vi "demod_low.vi"(0 "Reset":bool, 5 "Config":T5={"I/O"={"Format"={"Rate"=4, "Bits"=32, "Channels"=2}, "card #"=1, "# buffers"=96000}, "High rate STFT"={"Win param"=101.5, "Window type"=61, "Win order"=2, "DFT size"=64, "Channels"=[7], "Oversample"=64}, "Low rate STFT"={"Win param"=120.0, "Window type"=61, "Win order"=8, "DFT size"=64, "Channels"=[7], "Oversample"=64}, "Filtering"={"Hum"={"Frequency"=0.0, "Tc"=0.0, "Limit"=101.5, "FFT filter"=FALSE, "Detrend mode"=enum."Robust linear", "Enable"=FALSE}, "Kalman"={"Process noise"=101.5, "Measure noise"=101.5, "Unlock m noise"=101.5, "Mode"=enum."FFT"}, "Distortion"={"LF cut"=101.5, "Tc"=3.0, "Limit"=101.5, "FFT filter"=FALSE, "Detrend mode"=enum."Robust linear", "Enable"=FALSE}, "Lowpass"={"Frequency"=0.0, "Order"=0, "Enable"=FALSE}, "Impulse"={"Win order"=102, "Locked limit"=101.5, "Locked count"=102, "Threshold Tc"=101.5, "Thresh sigmas"=101.5, "Thresh min"=101.5, "After"=0, "Detrend"=FALSE, "Enable"=FALSE}}} {"Filtering"."Impulse"."Thresh min" format="%#_3p"; "Filtering"."Impulse"."Threshold Tc" format="%#_3p"; "Filtering"."Impulse"."Locked limit" format="%#_3p"; "Filtering"."Impulse"."Thresh sigmas" format="%#_3p"; "Filtering"."Lowpass"."Frequency" format="%#_4p"; "Filtering"."Distortion"."Limit" format="%#_3p"; "Filtering"."Distortion"."LF cut" format="%#_3p"; "Filtering"."Kalman"."Unlock m noise" format="%#_3p"; "Filtering"."Kalman"."Measure noise" format="%#_3p"; "Filtering"."Kalman"."Process noise" format="%#_3p"; "Filtering"."Hum"."Limit" format="%#_3p"; "Filtering"."Hum"."Frequency" format="%#_4p"; "Low rate STFT"."Oversample" min=1 step=1; "Low rate STFT"."Channels" min=0 step=1; "Low rate STFT"."DFT size" min=1 step=1; "Low rate STFT"."Window type" items=["Rectangle"=0, "Hanning"=1, "Hamming"=2, "Blackman-Harris"=3, "Exact Blackman"=4, "Blackman"=5, "Flat Top"=6, "4 Term B-Harris "=7, "7 Term B-Harris"=8, "Low Sidelobe"=9, "Blackman Nuttall"=11, "Triangle"=30, "Bartlett-Hanning"=31, "Bohman"=32, "Parzen"=33, "Welch"=34, "Kaiser"=60, "Dolph-Chebyshev"=61, "Gaussian"=62]; "High rate STFT"."Oversample" min=1 step=1; "High rate STFT"."Channels" min=0 step=1; "High rate STFT"."DFT size" min=1 step=1; "High rate STFT"."Window type" items=["Rectangle"=0, "Hanning"=1, "Hamming"=2, "Blackman-Harris"=3, "Exact Blackman"=4, "Blackman"=5, "Flat Top"=6, "4 Term B-Harris "=7, "7 Term B-Harris"=8, "Low Sidelobe"=9, "Blackman Nuttall"=11, "Triangle"=30, "Bartlett-Hanning"=31, "Bohman"=32, "Parzen"=33, "Welch"=34, "Kaiser"=60, "Dolph-Chebyshev"=61, "Gaussian"=62]}, 7 "Modulation info":T1={"Fs full"=0.0, "Fs high"=0.0, "Fs low"=0.0, "Read size"=0, "FFT size low"=5000, "df low"=5000.0, "High carriers"=[], "Low carriers"=[], "Hi channels at low"=[7]} {"Hi channels at low" min=0 step=1; "Low carriers" format="%#_6p"; "High carriers" format="%#_6p"}, 11 "Trace info in":T2, 12 "Filtered data":dbl[][](array[numeric])) -> (4 "Carrier amplitudes":cdb[][][](array[numeric]) format="%#_3p", 15 "Trace info out":T2)   [LabVIEW 2014]
uses:
  ilemt_config.ctl
  io_config.ctl
  stft_params.ctl
  <vilib>/Analysis/4window.llb/windowTd.ctl
  filter_params.ctl
  detrend_mode.ctl
  trace_info.ctl
  trace_channel.ctl
  ilemt_status.ctl
  modulation_info.ctl
  <vilib>/Analysis/NI_AALPro.lvlib
panel:
  # "Rows are same format as raw data, 3 filtered sensor signals, followed by 3 (not Kalman filtered) current sense inputs."
  # "First dimension (page) selects input channel: sensor X, Y, Z or current sense.  There is only one set of currents even though there are three sense inputs because we only report X magnitude on X, Y on Y, etc., discarding the cross coupling terms."
  # "High"
  # "Low"
  # "X"
  # "Y"
  # "Z"
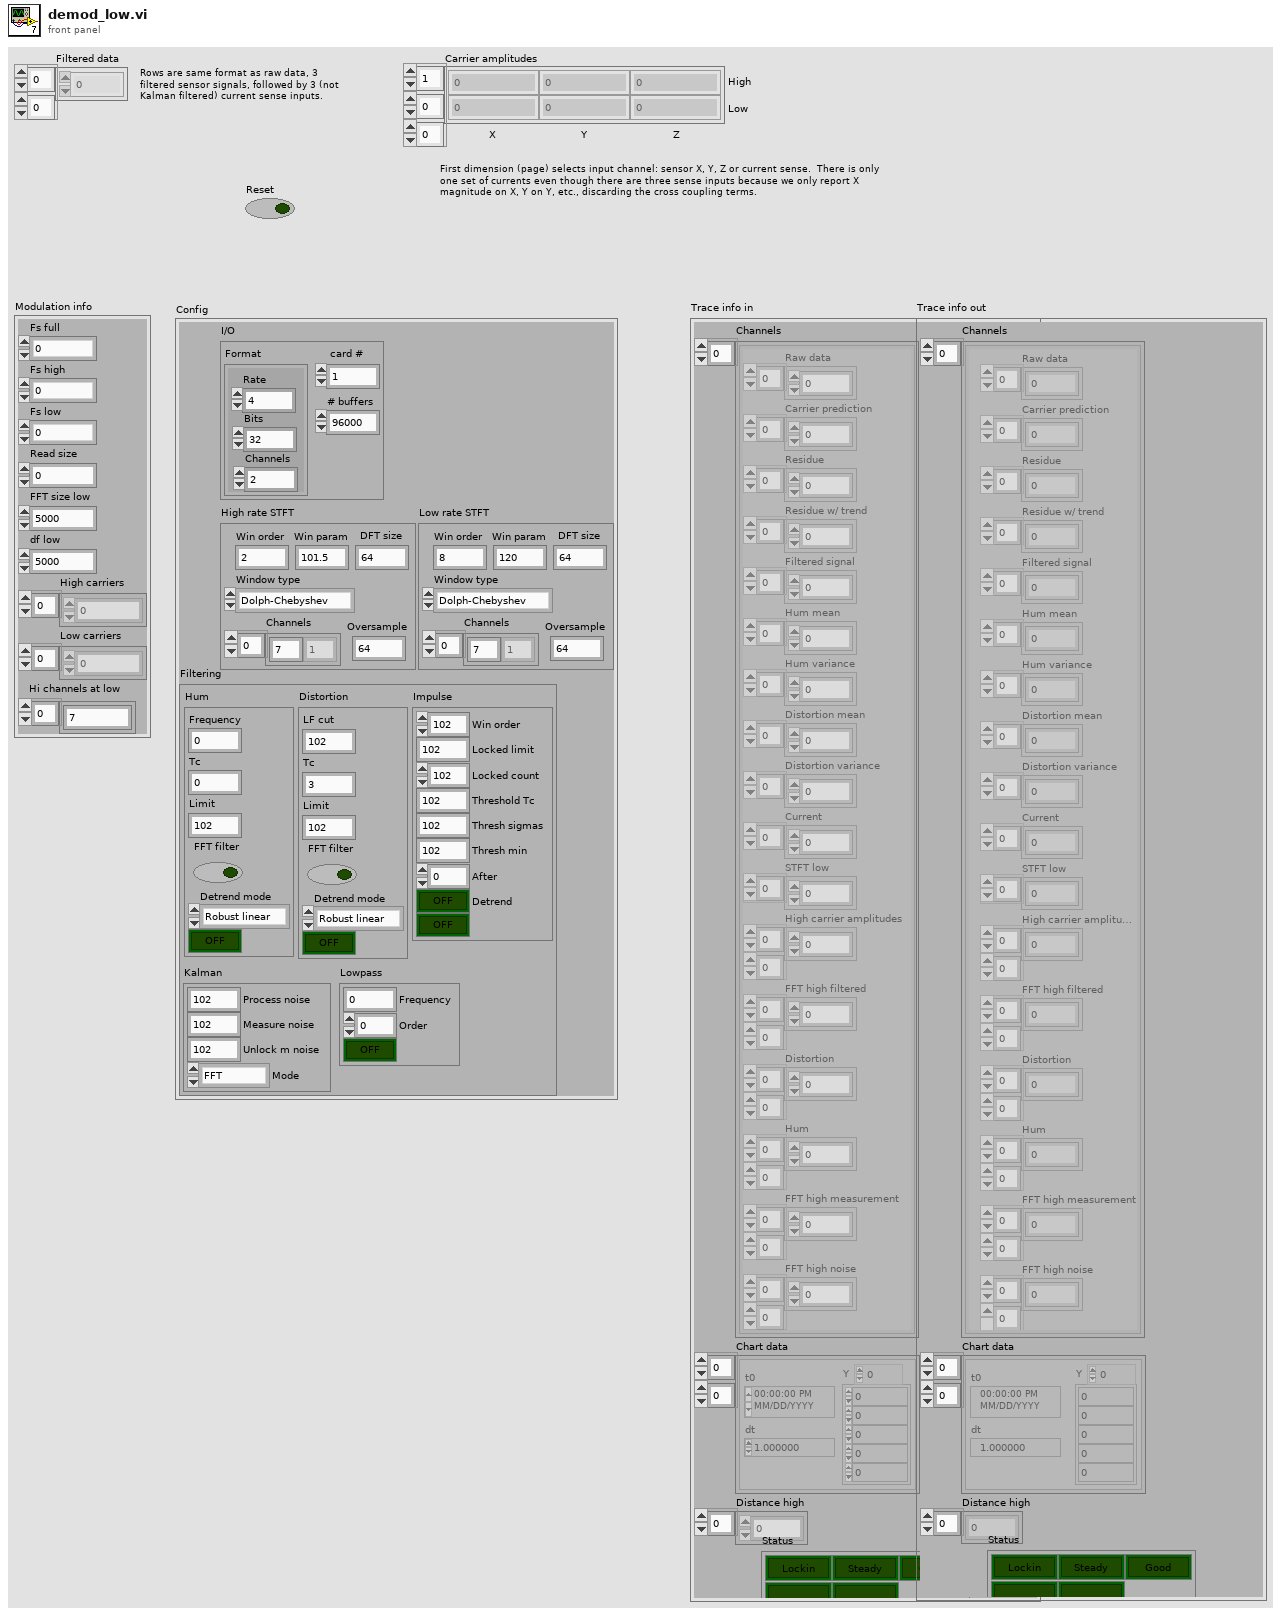
[diagram p1: front panel]
types:
  T1 = typedef "modulation_info.ctl" = cluster{"Fs full":dbl, "Fs high":dbl, "Fs low":dbl, "Read size":i32, "FFT size low":i32, "df low":dbl, "High carriers":dbl[], "Low carriers":dbl[], "Hi channels at low":i32[]}
  T2 = typedef "trace_info.ctl" = cluster{"Channels":T3[], "Chart data":waveform(dbl)[][], "Distance high":dbl[], "Status":T4}
  T3 = typedef "trace_channel.ctl" = cluster{"Raw data":dbl[], "Carrier prediction":dbl[], "Residue":dbl[], "Residue w/ trend":dbl[], "Filtered signal":dbl[], "Hum mean":dbl[], "Hum variance":dbl[], "Distortion mean":dbl[], "Distortion variance":dbl[], "Current":dbl[], "STFT low":cdb[], "High carrier amplitudes":cdb[][], "FFT high filtered":cdb[][], "Distortion":cdb[][], "Hum":cdb[][], "FFT high measurement":cdb[][], "FFT high noise":dbl[][]}
  T4 = typedef "ilemt_status.ctl" = cluster{"Unlocked":bool, "Impulse":bool, "NaN":bool, "Backlog":bool, "Clipping":bool}
  T5 = typedef "ilemt_config.ctl" = cluster{"I/O":T6, "High rate STFT":T7, "Low rate STFT":T7, "Filtering":T9}
  T6 = typedef "io_config.ctl" = cluster{"Format":cluster{"Rate":i32, "Bits":i32, "Channels":u32}, "card #":u32, "# buffers":i32}
  T7 = typedef "stft_params.ctl" = cluster{"Win param":dbl, "Window type":T8, "Win order":i32, "DFT size":i32, "Channels":i32[], "Oversample":i32}
  T8 = typedef "NI_AALPro.lvlib/windowTd.ctl" = u32
  T9 = typedef "filter_params.ctl" = cluster{"Hum":cluster{"Frequency":dbl, "Tc":dbl, "Limit":dbl, "FFT filter":bool, "Detrend mode":T10, "Enable":bool}, "Kalman":cluster{"Process noise":dbl, "Measure noise":dbl, "Unlock m noise":dbl, "Mode":enum16{"FFT", "KF demod"}}, "Distortion":cluster{"LF cut":dbl, "Tc":dbl, "Limit":dbl, "FFT filter":bool, "Detrend mode":T10, "Enable":bool}, "Lowpass":cluster{"Frequency":dbl, "Order":i32, "Enable":bool}, "Impulse":cluster{"Win order":i32, "Locked limit":dbl, "Locked count":i32, "Threshold Tc":dbl, "Thresh sigmas":dbl, "Thresh min":dbl, "After":i32, "Detrend":bool, "Enable":bool}}
  T10 = typedef "detrend_mode.ctl" = enum16{"Zero mean", "Linear", "Robust linear"}
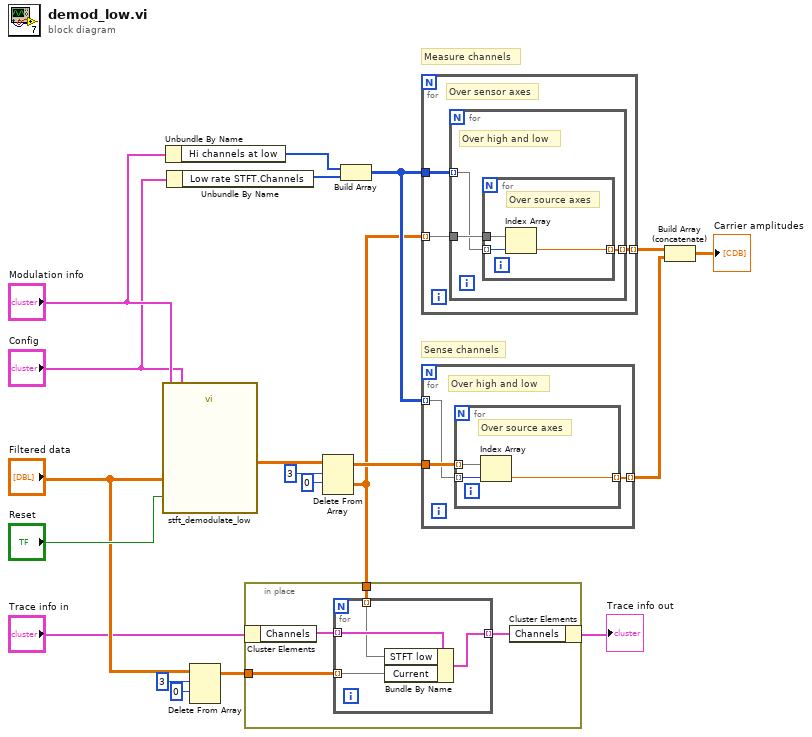
[diagram p0: block diagram]
diagram:
  # "Measure channels"
  # "Sense channels"
  n1 = call "stft_demodulate_low.vi"("Reset"="Reset", "Config"="Config", "Modulation info"="Modulation info", "Raw data"="Filtered data") -> ("STFT"=w12:cdb[][])  [unwired: 6 in, 1 out]
  n2 = Unbundle By Name("Modulation info") -> ("Hi channels at low"=w19:i32[])
  n3 = Unbundle By Name("Config") -> ("Low rate STFT.Channels"=w20:i32[])
  n4 = Delete From Array(array="Filtered data", length=3, index (row)=0) -> (array with subset deleted=w13:dbl[][])  [unwired: 1 in, 1 out]
  n5 = Delete From Array(array=w12, length=3, index (row)=0) -> (deleted portion=w2:cdb[][], array with subset deleted=w9:cdb[][])  [unwired: 1 in]
  n6 = in-place {
    in-place-border: w13 -> [w24]
    in-place-border: w2 -> [w22]
    n7 = in-place-cluster #1("Trace info in") -> ("Channels"=w23:T3[])
    n8 = for {
      tunnel: [w28] -> w21 mode=indexing
      tunnel: w24 -> [w27] mode=indexing
      tunnel: w23 -> [w26] mode=indexing
      tunnel: w22 -> [w25] mode=indexing
      n9 = Bundle By Name(cluster=w26, "STFT low"=w25, "Current"=w27) -> (w28:T3)
    }
    n10 = in-place-cluster #1("Channels"=w21) -> (→"Trace info out":T2)
  }
  n11 = Build Array(w19, w20) -> (w10:i32[][])
  n12 = for {
    tunnel: w10 -> [w31]
    tunnel: [w30] -> w8 mode=indexing
    tunnel: w2 -> [w29] mode=indexing
    # "Over sensor axes"
    n13 = for {
      tunnel: w29 -> [w34]
      tunnel: w31 -> [w33] mode=indexing
      tunnel: [w32] -> w30 mode=indexing
      # "Over high and low"
      n14 = for {
        tunnel: w34 -> [w37]
        tunnel: w33 -> [w35] mode=indexing
        tunnel: [w36] -> w32 mode=indexing
        # "Over source axes"
        n15 = Index Array(array=w37, index=w35) -> (element=w36:cdb)
      }
    }
  }
  n16 = for {
    tunnel: w9 -> [w40]
    tunnel: w10 -> [w39] mode=indexing
    tunnel: [w38] -> w7 mode=indexing
    # "Over high and low"
    n17 = for {
      tunnel: w40 -> [w43] mode=indexing
      tunnel: w39 -> [w42] mode=indexing
      tunnel: [w41] -> w38 mode=indexing
      # "Over source axes"
      n18 = Index Array(array=w43, index=w42) -> (element=w41:cdb)
    }
  }
  n19 = Build Array (concatenate)(w8, w7) -> (→"Carrier amplitudes":cdb[][][])
